vi "Read I64.vi"(8 "error in (no error)":errorcluster, 11 "Event in":refnum<class "Event I64.lvclass">) -> (0 "error out":errorcluster, 2 "I64":i64, 3 "Event out":refnum<class "Event I64.lvclass">)   [LabVIEW 2023, in "MVC Actors.lvlib" / "Event I64.lvclass"]
uses:
  Event I64.lvclass
  Event I64.lvclass/Event I64.ctl
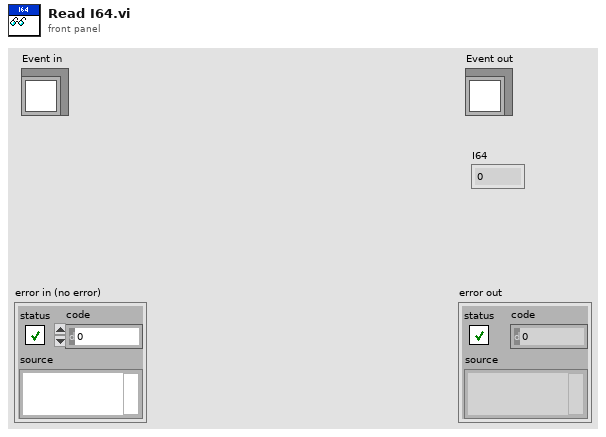
[diagram p1: front panel]
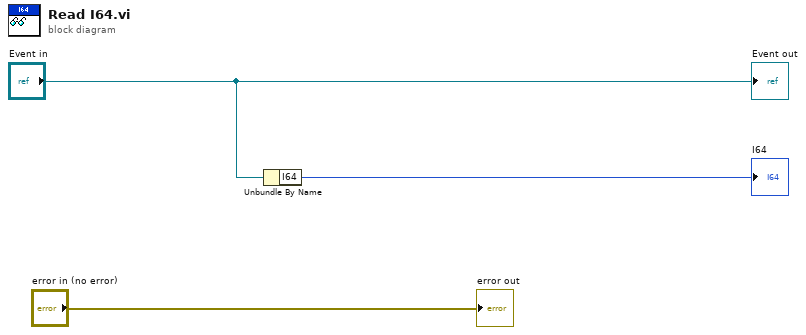
[diagram p0: block diagram]
diagram:
  n1 = Unbundle By Name("Event in") -> ("I64"=→"I64":i64)
  "Event out" <- "Event in"
  "error out" <- "error in (no error)"
